vi "update_last_id_ajuste_previo.vi"(8 "error in (no error)":errorcluster) -> (0 "error out":errorcluster, 3 "last_id_ajuste_previo":i32)   [LabVIEW 2019, in "Base de Datos.lvclass"]
uses:
  Base de Datos.lvclass
  Globals/globales.vi
  SQLiteConnector/SQLiteConnection.lvclass
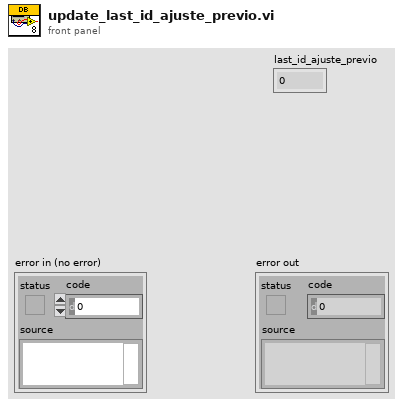
[diagram p1: front panel]
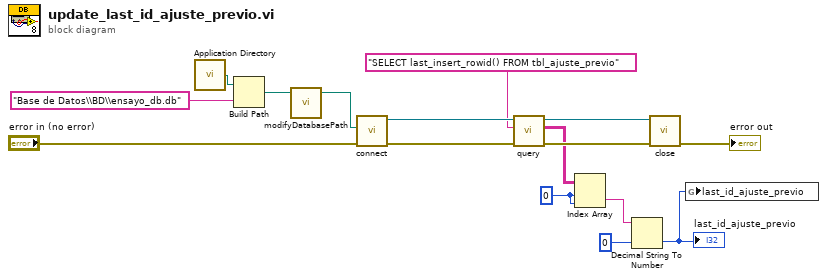
[diagram p0: block diagram]
diagram:
  w5 = 0 ("index (row)")
  n1 = call <vilib>:"Application Directory.vi"() -> ("Application Directory"=w16:path)
  n2 = Build Path(base path=w16, name or relative path="Base de Datos\\BD\\ensayo_db.db" ("BD")) -> (appended path=w15:path)
  n3 = call "modifyDatabasePath.vi"("Database Path In"=w15) -> ("Database Path Out"=w14:path)  [unwired: 4 in]
  n4 = call "connect.vi"("error in (no error)"="error in (no error)", "Database Path"=w14) -> ("error out"=w11:errorcluster, "object out"=w12:refnum<class "SQLiteConnection.lvclass">)  [unwired: 8 in]
  n5 = call "query.vi"("error in (no error)"=w11, "SQL Statement"="SELECT last_insert_rowid() FROM tbl_ajuste_previo" ("time format string (%c)"), "object in"=w12) -> ("error out"=w9:errorcluster, "result"=w6:string[][], "object out"=w8:refnum<class "SQLiteConnection.lvclass">)  [unwired: 5 in, 1 out]
  n6 = Index Array(array=w6, index (row)=w5, index (col)=w5) -> (element=w4:string)
  n7 = Decimal String To Number(string=w4, default (0L)=0) -> (number=w1:i32)  [unwired: 1 in, 1 out]
  "last_id_ajuste_previo" <- w1
  n8 = call-dynamic "close.vi"("error in (no error)"=w9, "object in"=w8) -> ("error out"=→"error out":errorcluster)  [unwired: 8 in, 1 out]
  n9 = global write "globales.vi" "last_id_ajuste_previo"(w1) -> ()
